vi "Configure GMaps Request.vi"(0 "GMaps API in":refnum<class "GMaps API.lvclass">, 1 "GMap Options":cluster{"URL":T1, "Path":T2, "Marker":T3} {"URL"."Zoom" items=["World"=1, "Landmass/continent"=5, "City"=10, "Street"=15, "Building"=20]}, 5 "error in (no error)":errorcluster) -> (14 "GMaps API out":refnum<class "GMaps API.lvclass">, 19 "error out":errorcluster)   [LabVIEW 2016, in "GMaps API.lvclass"]
doc: "Provides GMaps configuration options."
uses:
  GMaps API.lvclass
  Controls/URL.ctl
  Controls/Path.ctl
  Controls/Marker.ctl
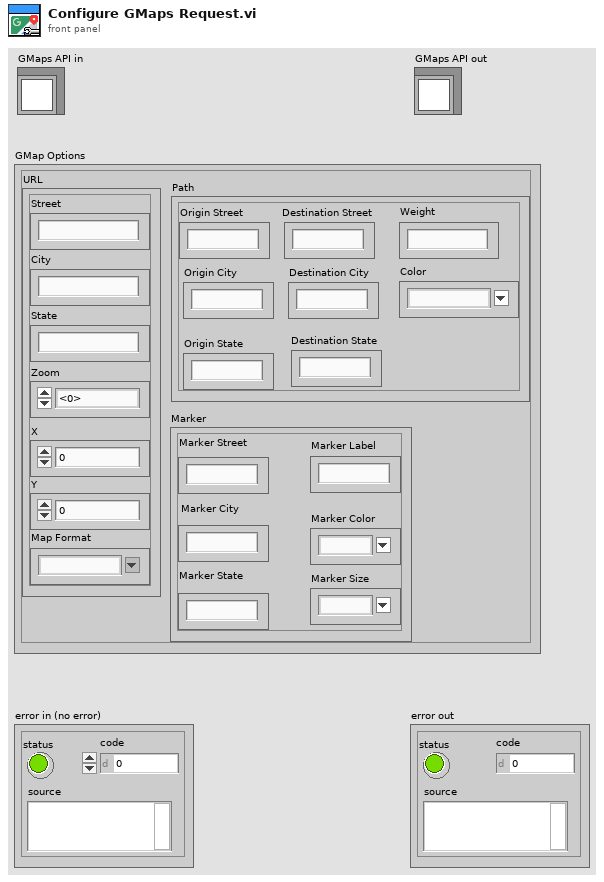
[diagram p1: front panel]
types:
  T1 = typedef "GMaps API.lvclass/URL.ctl" = cluster{"Street":string, "State":string, "City":string, "X":u32, "Y":u32, "Map Format":string, "Zoom":u64}
  T2 = typedef "GMaps API.lvclass/Path.ctl" = cluster{"Color":string, "Weight":string, "Destination State":string, "Destination City":string, "Destination Street":string, "Origin State":string, "Origin City":string, "Origin Street":string}
  T3 = typedef "GMaps API.lvclass/Marker.ctl" = cluster{"Marker Color":string, "Marker Size ":string, "Marker Label":string, "Marker State":string, "Marker City":string, "Marker Street":string}
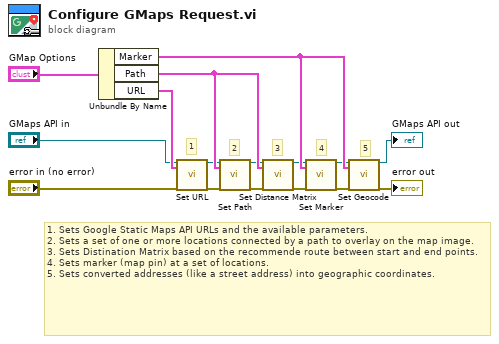
[diagram p0: block diagram]
diagram:
  # "5"
  # "4"
  # "3"
  # "2"
  # "1"
  # "1. Sets Google Static Maps API URLs and the available parameters.\n2. Sets a set of one or more locations connected by a path to overlay on the map image.\n3. Sets Distination Matrix based on the recommende route between start and end points.\n4. Sets marker (map pin) at a set of locations.\n5. Sets converted addresses (like a street address) into geographic coordinates."
  n1 = Unbundle By Name("GMap Options") -> ("Marker"=w14:T3, "Path"=w15:T2, "URL"=w16:T1)
  n2 = call "Set URL.vi"("GMaps API in"="GMaps API in", "URL"=w16, "error in (no error)"="error in (no error)") -> ("GMaps API out"=w5:refnum<class "GMaps API.lvclass">, "error out"=w6:errorcluster)  [unwired: 15 in]
  n3 = call "Set Path.vi"("GMaps API in"=w5, "Path"=w15, "error in (no error)"=w6) -> ("GMaps API out"=w8:refnum<class "GMaps API.lvclass">, "error out"=w7:errorcluster)  [unwired: 15 in]
  n4 = call "Set Distance Matrix.vi"("GMaps API in"=w8, "Path"=w15, "error in (no error)"=w7) -> ("GMaps API out"=w9:refnum<class "GMaps API.lvclass">, "error out"=w10:errorcluster)  [unwired: 15 in]
  n5 = call "Set Marker.vi"("GMaps API in"=w9, "Marker"=w14, "error in (no error)"=w10) -> ("GMaps API out"=w11:refnum<class "GMaps API.lvclass">, "error out"=w12:errorcluster)  [unwired: 15 in]
  n6 = call "Set Geocode.vi"("GMaps API in"=w11, "Marker"=w14, "error in (no error)"=w12) -> ("GMaps API out"=→"GMaps API out":refnum<class "GMaps API.lvclass">, "error out"=→"error out":errorcluster)  [unwired: 15 in]
